vi "Begin.vi"(11 "Image Size":T1=enum."160x120") -> (0 "error out":errorcluster)   [LabVIEW 2012]
doc: "Called before other user functions, this VI is expected to open initial I/O refnums, load in file data, and do all program initialization. Notice that the <B>error out</B> terminal is simply used for data flow. Wiring it to other structures or subVIs ensures that this VI runs first."
uses:
  <vilib>/Rock Robotics/WPI/Camera/WPI_CameraImageSize.ctl
  <vilib>/Rock Robotics/WPI/DriverStation/WPI_DriverStationRobotMode2.ctl
  <vilib>/Rock Robotics/WPI/CAN/Jaguar/SubVIs/WPI_CANJaguar_SpeedReference.ctl
  <vilib>/Rock Robotics/WPI/CAN/Jaguar/SubVIs/WPI_CANJaguar_ControlMode.ctl
  <vilib>/Rock Robotics/WPI/CAN/Jaguar/SubVIs/WPI_CANJaguar_BrakeCoastMode.ctl
  <vilib>/Rock Robotics/WPI/Joystick/WPI_JoystickDeviceEnum.ctl
  Robot Global Data.vi
  <vilib>/Rock Robotics/WPI/MotorControl/WPI_MotorControlOpenCANJaguar.vi
  <vilib>/Rock Robotics/WPI/RobotDrive/WPI_RobotDriveOpen2MotorWithJaguar.vi
  <vilib>/Rock Robotics/SystemInterfaces/DIO/FPGA_DIOPWMChannel.ctl
  <vilib>/Rock Robotics/WPI/Camera/WPI_CameraWhite Balance Values.ctl
  <vilib>/Rock Robotics/WPI/Camera/WPI_CameraExposure Values.ctl
  <vilib>/Rock Robotics/WPI/Camera/WPI_CameraFrameRate.ctl
  <vilib>/Rock Robotics/WPI/SafetyOutput/WPI_SafetyOutputConfigMenu.ctl
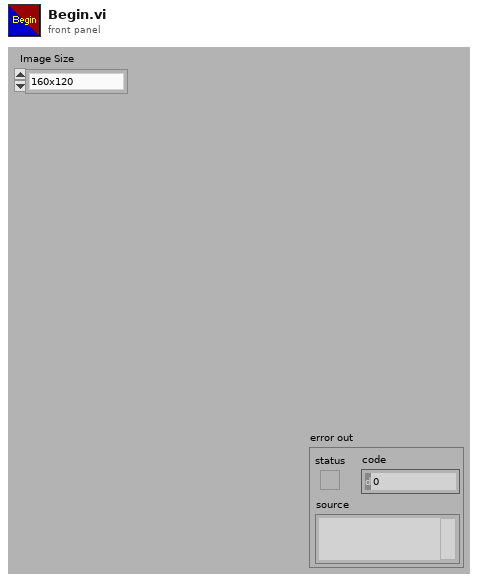
[diagram p1: front panel]
types:
  T1 = typedef "WPI_CameraImageSize.ctl" = enum16{"640x480", "320x240", "160x120"}
  T2 = typedef "WPI_JoystickDeviceEnum.ctl" = enum16{"USB 1", "USB 2", "USB 3", "USB 4", "Kinect 1", "Kinect 2"}
  T3 = typedef "WPI_CANJaguar_BrakeCoastMode.ctl" = enum8{"Jumper", "Brake", "Coast"}
  T4 = typedef "WPI_CANJaguar_SpeedReference.ctl" = u8
  T5 = typedef "WPI_CANJaguar_ControlMode.ctl" = enum8{"Percent VBus", "Current", "Speed", "Position", "Voltage"}
  T6 = typedef "WPI_DriverStationRobotMode2.ctl" = enum16{"Autonomous Disabled", "Autonomous Enabled", "Teleop Disabled", "Teleop Enabled", "Timeout", "Finish", "Test Disabled", "Test Enabled"}
  T7 = typedef "WPI_JoystickDevRef.ctl" = cluster{"Device":T2}
  T8 = typedef "WPI_CameraFrameRate.ctl" = u32
  T9 = typedef "WPI_CameraExposure Values.ctl" = enum16{"Auto", "Flicker-free 50 Hz", "Flicker-free 60 Hz", "Hold current"}
  T10 = typedef "WPI_CameraWhite Balance Values.ctl" = enum16{"Auto", "Fixed indoor", "Fixed outdoor 1", "Fixed outdoor 2", "Fixed fluorescent 1", "Fixed fluorescent 2", "Hold current"}
  T11 = typedef "WPI_CameraDevRef.ctl" = cluster{"Camera Address":string, "CameraStatus":errorcluster, "Acquire Image Notifier":refnum<notifier>}
  T12 = typedef "WPI_SafetyOutputConfigMenu.ctl" = enum16{"Enable", "Disable"}
  T13 = typedef "FPGA_DIOPWMChannel.ctl" = enum8{"PWM 1", "PWM 2", "PWM 3", "PWM 4", "PWM 5", "PWM 6", "PWM 7", "PWM 8", "PWM 9", "PWM 10", "Invalid"}
  T14 = typedef "WPI_RobotDriveDevRef.ctl" = cluster{"DevStatus":errorcluster, "Motors[]":T15[], "Square Inputs":bool, "Max Output":dbl, "Isochronous":bool}
  T15 = typedef "WPI_MotorControlDeviceRef.ctl" = cluster{"DeviceStatus":errorcluster, "Type":enum16{"PWM", "CAN"}, "PWM":cluster{"Digital Module":T16, "PWM Channel":T13, "DeadBand":T17}, "CAN":cluster{"Device Number":u8, "Control Mode":T5, "Semaphore":T18, "Max Vout":dbl}, "Invert":bool, "TransformRef":T19, "InvTransformRef":T19}
  T16 = typedef "FPGA_TypedefDigitalModule.ctl" = enum16{"Digital Module 1", "Digital Module 2"}
  T17 = typedef "WPI_PWMDeadband.ctl" = cluster{"Name":string, "maxPositivePwm":i32, "minPositivePwm":i32, "centerPwm":i32, "maxNegativePwm":i32, "minNegativePwm":i32, "angularRange":u16}
  T18 = typedef "Semaphore RefNum" = refnum<k1>
  T19 = typedef "WPI_PWMTransform_ConPane.ctl" = refnum<vi>
  T20 = typedef "WPI_SerialPortRef.ctl" = cluster{"DevStatus":errorcluster, "Serial Port Name":refnum<visa-resource-name>}
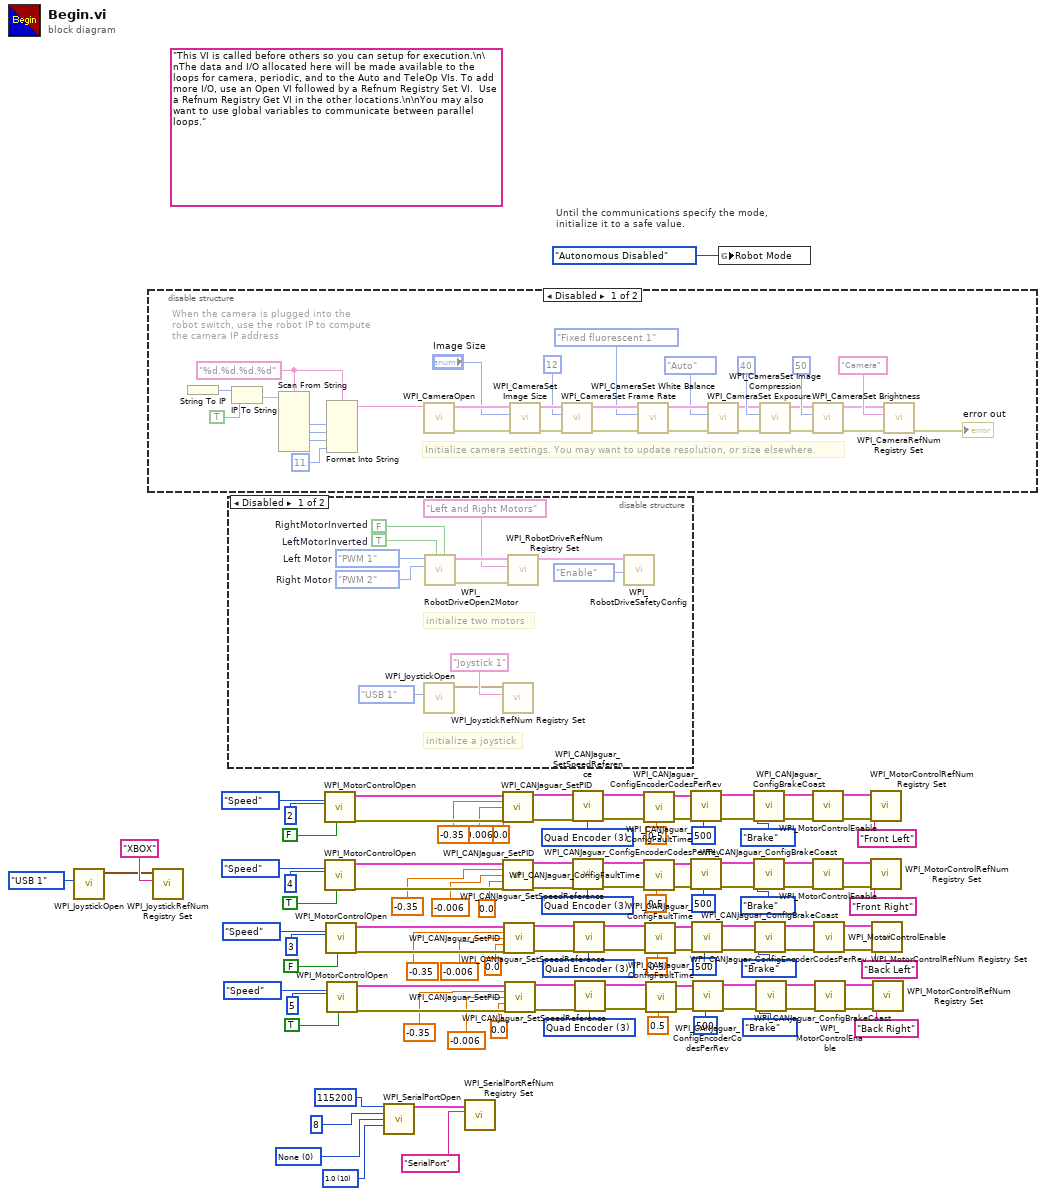
[diagram p0: block diagram]
diagram:
  w3 = u16 10 items=["1.0"=10, "1.5"=15, "2.0"=20] ("Stop Bits")
  w4 = u16 0 items=["None", "Odd", "Even", "Mark", "Space"] ("Parity")
  w30 = T4 3 items=["Encoder"=0, "Inv Encoder"=2, "Quad Encoder"=3, "None"=255] ("Speed Reference")
  w52 = T4 3 items=["Encoder"=0, "Inv Encoder"=2, "Quad Encoder"=3, "None"=255] ("Speed Reference")
  w74 = T4 3 items=["Encoder"=0, "Inv Encoder"=2, "Quad Encoder"=3, "None"=255] ("Speed Reference")
  w99 = T4 3 items=["Encoder"=0, "Inv Encoder"=2, "Quad Encoder"=3, "None"=255] ("Speed Reference")
  (unwired) "This VI is called before others so you can setup for execution.\n\nThe data and I/O allocated here will be made available to the loops for camera, periodic, and to the Auto and TeleOp VIs. To add more I/O, use an Open VI followed by a Refnum Registry Set VI.  Use a Refnum Registry Get VI in the other locations.\n\nYou may also want to use global variables to communicate between parallel loops."
  # "Until the communications specify the mode,\ninitialize it to a safe value."
  n1 = call <vilib>:"WPI_JoystickOpen.vi"("JoystickDevice"=WPI_JoystickDeviceEnum."USB 1") -> ("JoystickDevRef"=w17:T7)  [unwired: 10 in]
  n2 = disable-structure shown="Disabled" {
    frame Disabled {
      w113 = "%d.%d.%d.%d" ("format string")
      # "When the camera is plugged into the\nrobot switch, use the robot IP to compute\nthe camera IP address"
      # "Initialize camera settings. You may want to update resolution, or size elsewhere."
      n3 = String To IP() -> (0:w120:u32)  [unwired: 1 in]
      n4 = IP To String(1:TRUE ("dot notation? (F)"), 2:w120) -> (0:w118:string)
      n5 = Scan From String(format string=w113, input string=w118) -> (output 1=w117:i32, output 2=w116:i32, output 3=w115:i32)  [unwired: 7 in, 3 out]
      n6 = Format Into String(format string=w113, w117, w116, w115, 11 ("Compression")) -> (resulting string=w112:string)  [unwired: 2 in, 1 out]
      n7 = call <vilib>:"WPI_CameraOpen.vi"("Camera Address"=w112) -> ("error out"=w132:errorcluster, "CameraDevRef"=w133:T11)  [unwired: 1 in, 8 out]
      n8 = call <vilib>:"WPI_CameraSet Image Size.vi"("error in (no error)"=w132, "Image Size"="Image Size", "CameraDevRef"=w133) -> ("error out"=w131:errorcluster, "CameraDevRef Out"=w134:T11)  [unwired: 7 out]
      n9 = call <vilib>:"WPI_CameraSet Frame Rate.vi"("error in (no error)"=w131, "Frame Rate (fps)"=T8 12, "CameraDevRef"=w134) -> ("error out"=w130:errorcluster, "CameraDevRef Out"=w136:T11)  [unwired: 7 out]
      n10 = call <vilib>:"WPI_CameraSet White Balance.vi"("error in (no error)"=w130, "White Balance"=WPI_CameraWhite_Balance_Values."Fixed fluorescent 1", "CameraDevRef"=w136) -> ("error out"=w129:errorcluster, "CameraDevRef Out"=w135:T11)  [unwired: 7 out]
      n11 = call <vilib>:"WPI_CameraSet Exposure.vi"("error in (no error)"=w129, "Exposure"=WPI_CameraExposure_Values."Auto", "CameraDevRef"=w135) -> ("error out"=w128:errorcluster, "CameraDevRef Out"=w138:T11)  [unwired: 7 out]
      n12 = call <vilib>:"WPI_CameraSet Image Compression.vi"("error in (no error)"=w128, "Compression"=40, "CameraDevRef"=w138) -> ("error out"=w127:errorcluster, "CameraDevRef Out"=w137:T11)  [unwired: 7 out]
      n13 = call <vilib>:"WPI_CameraSet Brightness.vi"("error in (no error)"=w127, "Brightness"=50, "CameraDevRef"=w137) -> ("error out"=w125:errorcluster, "CameraDevRef Out"=w126:T11)  [unwired: 7 out]
      n14 = call <vilib>:"WPI_CameraRefNum Registry Set.vi"("error in (no error)"=w125, "refnum name"="Camera", "CameraDevRef"=w126) -> ("error out"=→"error out":errorcluster)  [unwired: 8 out]
    }
    frame Enabled {
    }
  }
  n15 = call <vilib>:"WPI_JoystickRefNum Registry Set.vi"("refnum name"="XBOX", "JoystickDevRef"=w17) -> ()  [unwired: 8 in, 2 out]
  n16 = disable-structure shown="Disabled" {
    frame Disabled {
      w147 = FPGA_DIOPWMChannel."PWM 2"  # Right Motor
      w148 = FPGA_DIOPWMChannel."PWM 1"  # Left Motor
      w152 = TRUE  # LeftMotorInverted
      w153 = FALSE  # RightMotorInverted
      # "initialize a joystick"
      # "initialize two motors"
      n17 = call <vilib>:"WPI_JoystickOpen.vi"("JoystickDevice"=WPI_JoystickDeviceEnum."USB 1") -> ("JoystickDevRef"=w143:T7)  [unwired: 10 in]
      n18 = call-poly <vilib>:"WPI_RobotDriveOpen2Motor.vi"("Right Motor Inverted"=w153, "Left Motor Inverted"=w152, "Right Motor"=w147, "Left Motor"=w148) -> ("error out"=w149:errorcluster, "RobotDriveDevRef"=w151:T14)  [unwired: 1 in, 5 out]
      n19 = call <vilib>:"WPI_JoystickRefNum Registry Set.vi"("refnum name"="Joystick 1", "JoystickDevRef"=w143) -> ()  [unwired: 8 in, 2 out]
      n20 = call <vilib>:"WPI_RobotDriveRefNum Registry Set.vi"("error in (no error)"=w149, "refnum name"="Left and Right Motors", "RobotDriveDevRef"=w151) -> ("RobotDriveDevRef"=w146:T14)  [unwired: 8 out]
      n21 = call <vilib>:"WPI_RobotDriveSafetyConfig.vi"("mode"=WPI_SafetyOutputConfigMenu."Enable", "RobotDriveDevRef"=w146) -> ()  [unwired: 8 in, 2 out]
    }
    frame Enabled {
    }
  }
  n22 = call-poly <vilib>:"WPI_MotorControlOpen.vi"("Invert"=FALSE, "Device Number"=u8 2, "Control Mode"=WPI_CANJaguar_ControlMode."Speed") -> ("error out"=w103:errorcluster, "MotorControlDeviceRef"=w102:T15)  [unwired: 7 in]
  n23 = call-poly <vilib>:"WPI_MotorControlOpen.vi"("Invert"=TRUE, "Device Number"=u8 4, "Control Mode"=WPI_CANJaguar_ControlMode."Speed") -> ("error out"=w78:errorcluster, "MotorControlDeviceRef"=w77:T15)  [unwired: 7 in]
  n24 = call-poly <vilib>:"WPI_MotorControlOpen.vi"("Invert"=FALSE, "Device Number"=u8 3, "Control Mode"=WPI_CANJaguar_ControlMode."Speed") -> ("error out"=w56:errorcluster, "MotorControlDeviceRef"=w55:T15)  [unwired: 7 in]
  n25 = call-poly <vilib>:"WPI_MotorControlOpen.vi"("Invert"=TRUE, "Device Number"=u8 5, "Control Mode"=WPI_CANJaguar_ControlMode."Speed") -> ("error out"=w34:errorcluster, "MotorControlDeviceRef"=w33:T15)  [unwired: 7 in]
  n26 = call <vilib>:"WPI_SerialPortOpen.vi"("Baud Rate"=u32 115200, "Data Bits"=u16 8, "Parity"=w4, "Stop Bits"=w3) -> ("SerialPortRef"=w2:T20)  [unwired: 10 in, 1 out]
  n27 = call <vilib>:"WPI_SerialPortRefNum Registry Set.vi"("refnum name"="SerialPort", "SerialPortRef"=w2) -> ()  [unwired: 8 in, 2 out]
  n28 = call <vilib>:"WPI_CANJaguar_SetPID.vi"("CAN Jaguar Ref"=w102, "P"=-0.35, "I"=-0.006, "D"=0.0, "error in (no error)"=w103) -> ("CAN Jaguar Ref Out"=w109:T15, "error out"=w108:errorcluster)  [unwired: 9 in]
  n29 = call <vilib>:"WPI_CANJaguar_SetPID.vi"("CAN Jaguar Ref"=w77, "P"=-0.35, "I"=-0.006, "D"=0.0, "error in (no error)"=w78) -> ("CAN Jaguar Ref Out"=w84:T15, "error out"=w83:errorcluster)  [unwired: 9 in]
  n30 = call <vilib>:"WPI_CANJaguar_SetPID.vi"("CAN Jaguar Ref"=w55, "P"=-0.35, "I"=-0.006, "D"=0.0, "error in (no error)"=w56) -> ("CAN Jaguar Ref Out"=w62:T15, "error out"=w61:errorcluster)  [unwired: 9 in]
  n31 = call <vilib>:"WPI_CANJaguar_SetPID.vi"("CAN Jaguar Ref"=w33, "P"=-0.35, "I"=-0.006, "D"=0.0, "error in (no error)"=w34) -> ("CAN Jaguar Ref Out"=w40:T15, "error out"=w39:errorcluster)  [unwired: 9 in]
  n32 = call <vilib>:"WPI_CANJaguar_SetSpeedReference.vi"("error in (no error)"=w108, "Speed Reference"=w99, "CAN Jaguar Ref"=w109) -> ("error out"=w107:errorcluster, "CAN Jaguar Ref Out"=w106:T15)  [unwired: 7 in]
  n33 = call <vilib>:"WPI_CANJaguar_SetSpeedReference.vi"("error in (no error)"=w83, "Speed Reference"=w74, "CAN Jaguar Ref"=w84) -> ("error out"=w82:errorcluster, "CAN Jaguar Ref Out"=w81:T15)  [unwired: 7 in]
  n34 = call <vilib>:"WPI_CANJaguar_SetSpeedReference.vi"("error in (no error)"=w61, "Speed Reference"=w52, "CAN Jaguar Ref"=w62) -> ("error out"=w60:errorcluster, "CAN Jaguar Ref Out"=w59:T15)  [unwired: 7 in]
  n35 = call <vilib>:"WPI_CANJaguar_SetSpeedReference.vi"("error in (no error)"=w39, "Speed Reference"=w30, "CAN Jaguar Ref"=w40) -> ("error out"=w38:errorcluster, "CAN Jaguar Ref Out"=w37:T15)  [unwired: 7 in]
  n36 = call <vilib>:"WPI_CANJaguar_ConfigFaultTime.vi"("error in (no error)"=w107, "Fault Time (s)"=0.5, "CAN Jaguar Ref"=w106) -> ("error out"=w104:errorcluster, "CAN Jaguar Ref Out"=w105:T15)  [unwired: 7 in]
  n37 = call <vilib>:"WPI_CANJaguar_ConfigFaultTime.vi"("error in (no error)"=w82, "Fault Time (s)"=0.5, "CAN Jaguar Ref"=w81) -> ("error out"=w79:errorcluster, "CAN Jaguar Ref Out"=w80:T15)  [unwired: 7 in]
  n38 = call <vilib>:"WPI_CANJaguar_ConfigFaultTime.vi"("error in (no error)"=w60, "Fault Time (s)"=0.5, "CAN Jaguar Ref"=w59) -> ("error out"=w57:errorcluster, "CAN Jaguar Ref Out"=w58:T15)  [unwired: 7 in]
  n39 = call <vilib>:"WPI_CANJaguar_ConfigFaultTime.vi"("error in (no error)"=w38, "Fault Time (s)"=0.5, "CAN Jaguar Ref"=w37) -> ("error out"=w35:errorcluster, "CAN Jaguar Ref Out"=w36:T15)  [unwired: 7 in]
  n40 = call <vilib>:"WPI_CANJaguar_ConfigEncoderCodesPerRev.vi"("error in (no error)"=w104, "Encoder Codes Per Rev"=u16 500, "CAN Jaguar Ref"=w105) -> ("error out"=w96:errorcluster, "CAN Jaguar Ref Out"=w95:T15)  [unwired: 7 in]
  n41 = call <vilib>:"WPI_CANJaguar_ConfigEncoderCodesPerRev.vi"("error in (no error)"=w79, "Encoder Codes Per Rev"=u16 500, "CAN Jaguar Ref"=w80) -> ("error out"=w71:errorcluster, "CAN Jaguar Ref Out"=w70:T15)  [unwired: 7 in]
  n42 = call <vilib>:"WPI_CANJaguar_ConfigEncoderCodesPerRev.vi"("error in (no error)"=w57, "Encoder Codes Per Rev"=u16 500, "CAN Jaguar Ref"=w58) -> ("error out"=w49:errorcluster, "CAN Jaguar Ref Out"=w48:T15)  [unwired: 7 in]
  n43 = call <vilib>:"WPI_CANJaguar_ConfigEncoderCodesPerRev.vi"("error in (no error)"=w35, "Encoder Codes Per Rev"=u16 500, "CAN Jaguar Ref"=w36) -> ("error out"=w27:errorcluster, "CAN Jaguar Ref Out"=w26:T15)  [unwired: 7 in]
  n44 = global write "Robot Global Data.vi" "Robot Mode"(WPI_DriverStationRobotMode2."Autonomous Disabled" ("Robot Mode")) -> ()
  n45 = call <vilib>:"WPI_CANJaguar_ConfigBrakeCoast.vi"("error in (no error)"=w96, "Brake / Coast Mode"=WPI_CANJaguar_BrakeCoastMode."Brake", "CAN Jaguar Ref"=w95) -> ("error out"=w87:errorcluster, "CAN Jaguar Ref Out"=w88:T15)  [unwired: 7 in]
  n46 = call <vilib>:"WPI_CANJaguar_ConfigBrakeCoast.vi"("error in (no error)"=w71, "Brake / Coast Mode"=WPI_CANJaguar_BrakeCoastMode."Brake", "CAN Jaguar Ref"=w70) -> ("error out"=w65:errorcluster, "CAN Jaguar Ref Out"=w66:T15)  [unwired: 7 in]
  n47 = call <vilib>:"WPI_CANJaguar_ConfigBrakeCoast.vi"("error in (no error)"=w49, "Brake / Coast Mode"=WPI_CANJaguar_BrakeCoastMode."Brake", "CAN Jaguar Ref"=w48) -> ("error out"=w43:errorcluster, "CAN Jaguar Ref Out"=w44:T15)  [unwired: 7 in]
  n48 = call <vilib>:"WPI_CANJaguar_ConfigBrakeCoast.vi"("error in (no error)"=w27, "Brake / Coast Mode"=WPI_CANJaguar_BrakeCoastMode."Brake", "CAN Jaguar Ref"=w26) -> ("error out"=w21:errorcluster, "CAN Jaguar Ref Out"=w22:T15)  [unwired: 7 in]
  n49 = call <vilib>:"WPI_MotorControlEnable.vi"("error in (no error)"=w87, "CAN Jaguar Ref"=w88) -> ("error out"=w85:errorcluster, "CAN Jaguar Ref Out"=w86:T15)  [unwired: 8 in]
  n50 = call <vilib>:"WPI_MotorControlEnable.vi"("error in (no error)"=w65, "CAN Jaguar Ref"=w66) -> ("error out"=w63:errorcluster, "CAN Jaguar Ref Out"=w64:T15)  [unwired: 8 in]
  n51 = call <vilib>:"WPI_MotorControlEnable.vi"("error in (no error)"=w43, "CAN Jaguar Ref"=w44) -> ("error out"=w41:errorcluster, "CAN Jaguar Ref Out"=w42:T15)  [unwired: 8 in]
  n52 = call <vilib>:"WPI_MotorControlEnable.vi"("error in (no error)"=w21, "CAN Jaguar Ref"=w22) -> ("error out"=w19:errorcluster, "CAN Jaguar Ref Out"=w20:T15)  [unwired: 8 in]
  n53 = call <vilib>:"WPI_MotorControlRefNum Registry Set.vi"("error in (no error)"=w85, "refnum name"="Front Left", "MotorControlDevRef"=w86) -> ()  [unwired: 7 in, 2 out]
  n54 = call <vilib>:"WPI_MotorControlRefNum Registry Set.vi"("error in (no error)"=w63, "refnum name"="Front Right", "MotorControlDevRef"=w64) -> ()  [unwired: 7 in, 2 out]
  n55 = call <vilib>:"WPI_MotorControlRefNum Registry Set.vi"("error in (no error)"=w41, "refnum name"="Back Left", "MotorControlDevRef"=w42) -> ()  [unwired: 7 in, 2 out]
  n56 = call <vilib>:"WPI_MotorControlRefNum Registry Set.vi"("error in (no error)"=w19, "refnum name"="Back Right", "MotorControlDevRef"=w20) -> ()  [unwired: 7 in, 2 out]
